vi "CalculateAlarms.vi"(6 "Settings":T1={"Name of test"="", "Date"=timestamp(0 s since 1904-01-01), "Location"="", "Template"="", "Soundcard"="", "resolution"=32, "Sampling rate"=48000, "Ch1 Gain "=25.0, "Ch2 Gain"=10.0, "Sample time (s)"=0.3, "Pre-trigger (s)"=0.01, "Hammer Threshold"=10.0, "Positions"=12, "Taps/Position"=5, "Set Names"="", "Freq resolution"=10.0, "Hammer cutoff"=0.0, "Mic cutoff"=0.0, "Double bounce "=0.0, "Hammer Cal"=10.0, "dB Offset"=0.0, "Accel Cal"=10.0, "Vibrometer Cal"=0.0, "Mic Cal"=0.0, "Output"=2, "Voltage Cal"=1.0, "Vibrometer Port"="ASRL27::INSTR", "Range"=4, "High Pass"=2, "Bandwidth"=4, "X Range"=[], "Y Range"=[], "dB Spread"=0.0, "Trigger"=0, "Ch_1"=25, "Ch_2"=25, "flip?"=FALSE, "60Hz"=FALSE, "Time offset"=0.0, "Piezo Cal"=1.0, "Default Notes"=""} {"Ch_2" min=1 step=1; "Ch_1" min=1 max=100 step=1; "Trigger" items=["Hammer (force)", "Self-tap", "Spacebar"]; "Bandwidth" items=["1 kHz"=1, "5 kHz"=5, "10 kHz"=10, "25 kHz"=25, "50 kHz"=50, "100 kHz"=100]; "High Pass" items=["Off", "13 Hz", "104 Hz"]; "Range" items=["10 mm/s"=1, "20 mm/s"=2, "50 mm/s"=5, "100 mm/s"=10, "200 mm/s"=20, "500 mm/s"=50, "1 m/s"=100, "2 m/s"=200]; "Output" items=["Accelerometer", "Speed (from acceleration)", "Microphone", "Vibrometer", "Piezo"]; "Voltage Cal" format="%#_13g"; "Ch2 Gain" format="%#_13g"; "Ch1 Gain" format="%#_13g"; "Double bounce" min=0.0; "Mic cutoff" min=0.0 format="%#_4g"; "Hammer cutoff" min=0.0 format="%#_4g"; "Freq resolution" min=0.0; "Pre-trigger (s)" format="%#_13g"; "Date" format="%<%H:%M\n%d/%m/%y>T"; "resolution" items=["16 bit"=16, "24 bit"=24, "32 bit"=32]; "Sampling rate" items=["22050 samp/s"=22050, "44100 samp/s"=44100, "48000 samp/s"=48000]}, 9 "last tap":waveform(dbl)[](array[waveform]), 10 "Last Path":path, 11 "Alarm":refnum<vi>) -> (1 "last tap?":bool, 3 "Good point?":bool)   [LabVIEW 2022 SP3]
uses:
  PreferencesControl.ctl
panel:
  out "String":string
  out "Alarm 2":string
  # "Hz"
  # "dB"
  # "dB"
  # "sec"
  # "sec"
  # "mV/Pa"
  # "mV/m/s2"
  # "mV/mm/s"
  # "V/N"
  # "sec"
  # "sec"
  # "mV/N"
  # "a.u."
  # "a.u."
  # "sec"
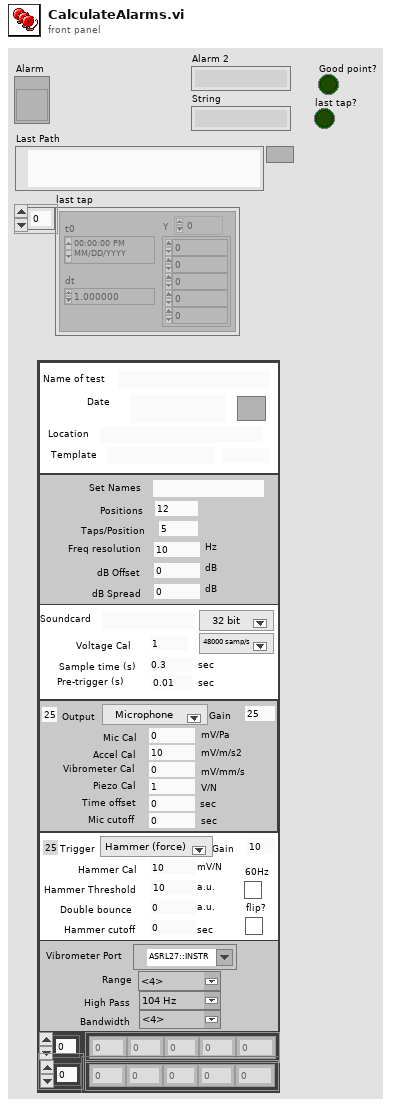
[diagram p1: front panel]
types:
  T1 = typedef "PreferencesControl.ctl" = cluster{"Name of test":string, "Date":timestamp, "Location":string, "Template":string, "Soundcard":string, "resolution":u16, "Sampling rate":u16, "Ch1 Gain ":dbl, "Ch2 Gain":dbl, "Sample time (s)":dbl, "Pre-trigger (s)":dbl, "Hammer Threshold":dbl, "Positions":i16, "Taps/Position":i16, "Set Names":string, "Freq resolution":dbl, "Hammer cutoff":dbl, "Mic cutoff":dbl, "Double bounce ":dbl, "Hammer Cal":dbl, "dB Offset":dbl, "Accel Cal":dbl, "Vibrometer Cal":dbl, "Mic Cal":dbl, "Output":u16, "Voltage Cal":dbl, "Vibrometer Port":refnum<visa-resource-name>, "Range":u16, "High Pass":u16, "Bandwidth":u16, "X Range":cluster{"Minimum":dbl, "Maximum":dbl, "Increment":dbl, "Minor Increment":dbl, "Start":dbl}[], "Y Range":cluster{"Minimum":dbl, "Maximum":dbl, "Increment":dbl, "Minor Increment":dbl, "Start":dbl}[], "dB Spread":dbl, "Trigger":u16, "Ch_1":u8, "Ch_2":u8, "flip?":bool, "60Hz":bool, "Time offset":dbl, "Piezo Cal":dbl, "Default Notes":string}
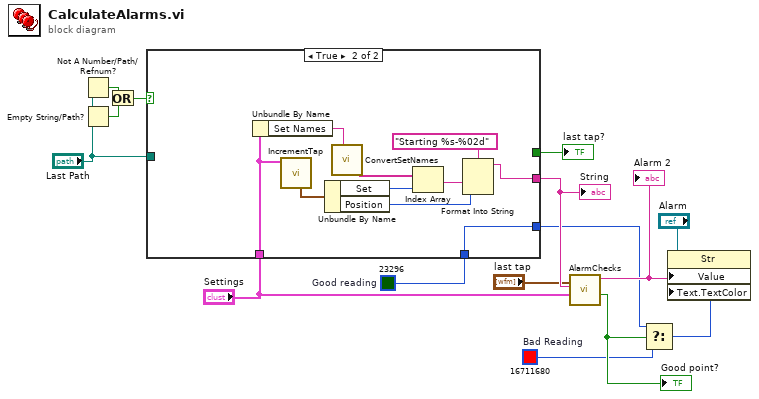
[diagram p0: block diagram]
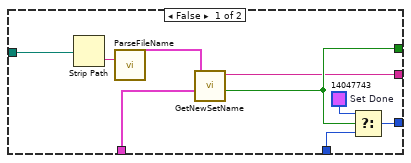
[diagram p2: hidden frame]
diagram:
  w3 = u32 23296  # Good reading
  w13 = u32 16711680  # Bad Reading
  n1 = Not A Number/Path/Refnum?(number/path/refnum="Last Path") -> (NaN/Path/Refnum?=w8:bool)
  n2 = Empty String/Path?(string/path="Last Path") -> (empty?=w7:bool)
  n3 = Or(x=w8, y=w7) -> (x .or. y?=w6:bool)
  n4 = case shown="True" w6 {
    tunnel: [w16 w32] -> w10
    tunnel: "Last Path" -> [w23 _]
    tunnel: "Settings" -> [w19 w30]
    tunnel: [w20 w25] -> w4
    tunnel: w3 -> [w21 w25]
    tunnel: [w17 _] -> w2
    frame False {
      w22 = u32 14047743  # Set Done
      n5 = Strip Path(path=w23) -> (name=w24:string)  [unwired: 1 out]
      n6 = call "ParseFileName.vi"("String in"=w24) -> ("Info"=w18:cluster{"Set":string, "Position":i32, "Tap":i32})  [unwired: 2 out]
      n7 = call "GetNewSetName.vi"("Settings"=w19, "Info"=w18) -> ("last tap?"=w17:bool, "String"=w16:string)  [unwired: 8 in]
      n8 = Select(t=w22, s=w17, f=w21) -> (s? t:f=w20:u32)
    }
    frame True {
      n9 = Unbundle By Name(w30) -> ("Set Names"=w29:string)
      n10 = call "IncrementTap.vi"("Settings"=w30) -> ("Location"=w34:cluster{"Set":i16, "Position":i16, "Tap":i16})  [unwired: 5 in, 5 out]
      n11 = Unbundle By Name(w34) -> ("Set"=w28:i16, "Position"=w33:i16)
      n12 = call "ConvertSetNames.vi"("Set Names"=w29) -> ("Set Names"=w27:string[])  [unwired: 10 in]
      n13 = Index Array(array=w27, index=w28) -> (element=w26:string)
      n14 = Format Into String(format string="Starting %s-%02d", w26, w33) -> (resulting string=w32:string)  [unwired: 2 in, 1 out]
    }
  }
  "last tap?" <- w2
  "String" <- w10
  n15 = call "AlarmChecks.vi"("Settings"="Settings", "Location"=w10, "last tap"="last tap") -> ("Good point?"=w15:bool, "Alarm"=w12:string)  [unwired: 7 in]
  "Good point?" <- w15
  "Alarm 2" <- w12
  n16 = Select(t=w4, s=w15, f=w13) -> (s? t:f=w14:u32)
  n17 = property class="Str"(reference="Alarm", "Value"=w12, "Text.TextColor"=w14) -> ()  [unwired: 1 in, 2 out]
